vi "温度扫描-热电偶.vi"(8 "error in (no error)":errorcluster, 9 "VISA resource name":refnum<visa-resource-name>="GPIB0::16::INSTR", 10 "Sample Count (100)":i32=100, 11 "Channel List (101:110)":string) -> (0 "error out":errorcluster, 3 "VISA resource name out":refnum<visa-resource-name>)   [LabVIEW 2020]
uses:
  <instrlib>/Keithley 27XX/Public/Configure/Measurement Specific/Configure Thermocouple.vi
  <instrlib>/Keithley 27XX/Keithley 27XX.lvlib
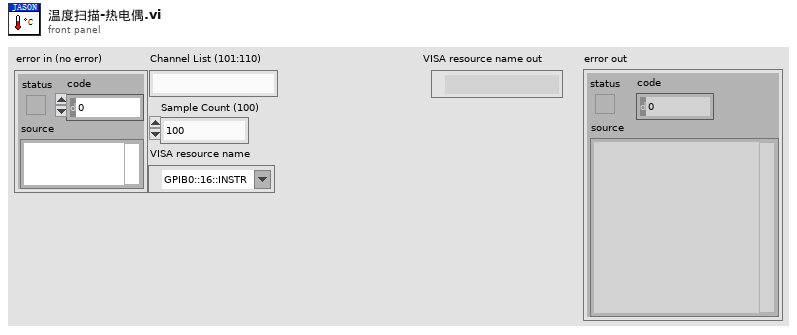
[diagram p1: front panel]
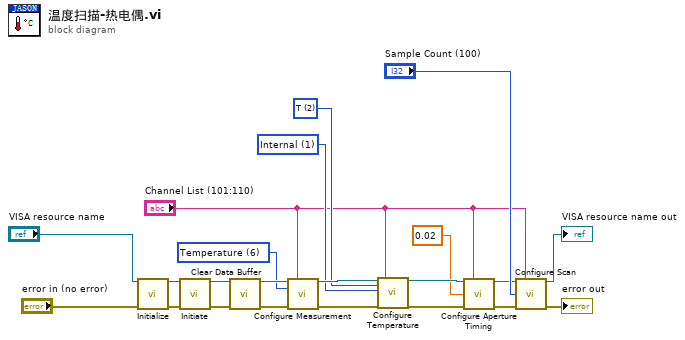
[diagram p0: block diagram]
diagram:
  w4 = u16 1 items=["Simulated", "Internal", "External"] ("Reference Junction Type (0: Simulated)")
  w5 = u16 2 items=["J", "K", "T", "E", "R", "S", "B", "N"] ("Thermocouple Type (1: K)")
  w21 = u16 6 items=["DC Voltage", "AC Voltage", "DC Current", "AC Current", "Resistance", "Four-Wire Resistance", "Temperature", "Frequency", "Period", "Continuity"] ("Function (0: DC Voltage)")
  n1 = call <instrlib>:"Initialize.vi"("VISA resource name"="VISA resource name", "error in (no error)"="error in (no error)") -> ("VISA resource name out"=w14:refnum<visa-resource-name>, "error out"=w12:errorcluster)  [unwired: 12 in]
  n2 = call <instrlib>:"Initiate.vi"("VISA resource name"=w14, "error in (no error)"=w12) -> ("VISA resource name out"=w13:refnum<visa-resource-name>, "error out"=w11:errorcluster)  [unwired: 12 in]
  n3 = call <instrlib>:"Clear Data Buffer.vi"("VISA resource name"=w13, "error in (no error)"=w11) -> ("VISA resource name out"=w22:refnum<visa-resource-name>, "error out"=w19:errorcluster)  [unwired: 12 in]
  n4 = call <instrlib>:"Configure Measurement.vi"("VISA resource name"=w22, "Scan List (Empty)"="Channel List (101:110)", "Function (0: DC Voltage)"=w21, "error in (no error)"=w19) -> ("VISA resource name out"=w20:refnum<visa-resource-name>, "error out"=w18:errorcluster)  [unwired: 10 in]
  n5 = call-poly <instrlib>:"Configure Temperature.vi"("VISA resource name"=w20, "Thermocouple Type (1: K)"=w5, "Reference Junction Type (0: Simulated)"=w4, "error in (no error)"=w18, "Scan List (Empty)"="Channel List (101:110)") -> ("VISA resource name out"=w7:refnum<visa-resource-name>, "error out"=w8:errorcluster)  [unwired: 13 in]
  n6 = call <instrlib>:"Configure Aperture Timing.vi"("VISA resource name"=w7, "Scan List (Empty)"="Channel List (101:110)", "Timing Value (0.020)"=0.02, "error in (no error)"=w8) -> ("VISA resource name out"=w2:refnum<visa-resource-name>, "error out"=w1:errorcluster)  [unwired: 10 in]
  n7 = call <instrlib>:"Configure Scan.vi"("VISA resource name"=w2, "Channel List (101:110)"="Channel List (101:110)", "Sample Count (100)"="Sample Count (100)", "error in (no error)"=w1) -> ("VISA resource name out"=→"VISA resource name out":refnum<visa-resource-name>, "error out"=→"error out":errorcluster)  [unwired: 10 in]
